vi "PCP Interface Loop.vi"(1 "PCP IO Loop ID":u16, 11 "error in (no error)":errorcluster) -> ()   [LabVIEW 2011]
uses:
  PCP Commands.ctl
  <vilib>/Instr/_visa.llb/VISA Flush IO Buffer Mask.ctl
  emi Lib/System 01/0 - General/App/Loop control 2/Private/_emi_ SMLoop start condition.vi
  emi Lib/System 01/0 - General/App/Loop control 2/Private/_emi_ SMLoop Error Check.vi
  emi Lib/Basic/0 - General/Error/emi_Is Error.vi
  emi Lib/System 01/0 - General/App/Loop control 2/Private/_emi_SMLoop Register new.vi
  emi Lib/System 01/0 - General/S&E reporting/emi_Send S&E Error message.vi
  emi Lib/Basic/0 - General/Error/emi_ Is Error state.vi
  emi Lib/System 01/0 - General/emi_Read System ID.vi
  emi Lib/System 01/0 - General/App/Loop control/Private/_emi_GFV Loop Linking.vi
  emi Lib/System 01/0 - General/App/Loop control/Private/_emi_GFV Loop Enable.vi
  emi Lib/System 01/0 - General/App/Loop control 2/Private/_emi_ SMLoop Restart.vi
  emi Lib/System 01/0 - General/App/Private/_emi_GFV App Close.vi
  emi Lib/System 01/0 - General/App/Loop control 2/Private/_emi_ SMLoop Restart Counter.vi
  emi Lib/System 01/0 - General/App/Loop control/Private/_emi_GFV Loop Running.vi
  emi Lib/System 01/0 - General/Private/_emi_GFV System ID.vi
  emi Lib/System 01/0 - General/S&E reporting/Private/_emi_S&E Q Generator.vi
  emi Lib/System 01/0 - General/App/Loop control/Private/_emi_GFV stop a loop so it can reset.vi
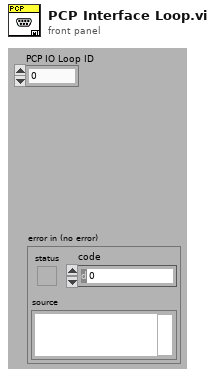
[diagram p1: front panel]
types:
  T1 = typedef "_emi_ SMLoop sates.ctl" = enum16{"Init", "Standby", "Start", "Normal Operation", "Stop", "Error Handling", "End", "Post"}
  T2 = cluster{"Placeholder":bool, "PCP cmd Q":refnum<queue>, "VISA name":refnum<visa-resource-name>}
  T3 = typedef "PCP Command definer.ctl" = cluster{"Action":T4, "n(0)":i32, "d(0.0)":dbl}
  T4 = typedef "PCP Commands.ctl" = enum16{"do not use HE - Help", "RDd - Most used inputs", "RA - All analog inputs", "RE n Reset DO n", "SE n Set DO n", "RP - Get digital inputs", "VA d Set AO A  Motor Volt", "VB d Set AO B  Cable Resistance", "VEr - Get Version", "DYp - Depth counter", "DR - Reset Depth Counter", "DS n Set Depth options(0-3)", "do not use ME - Manual mode enabled", "MD - Manual mode disabled", "ID - Get ID(2001)", "TS - Get Timestamp", "TO d(s)  Set timeout", "do not use LO n Start Loop Mode(1,2)", "AL n RD&LO variation", "ST - Stop Loop Mode"}
  T5 = typedef "VISA Flush IO Buffer Mask.ctl" = u16
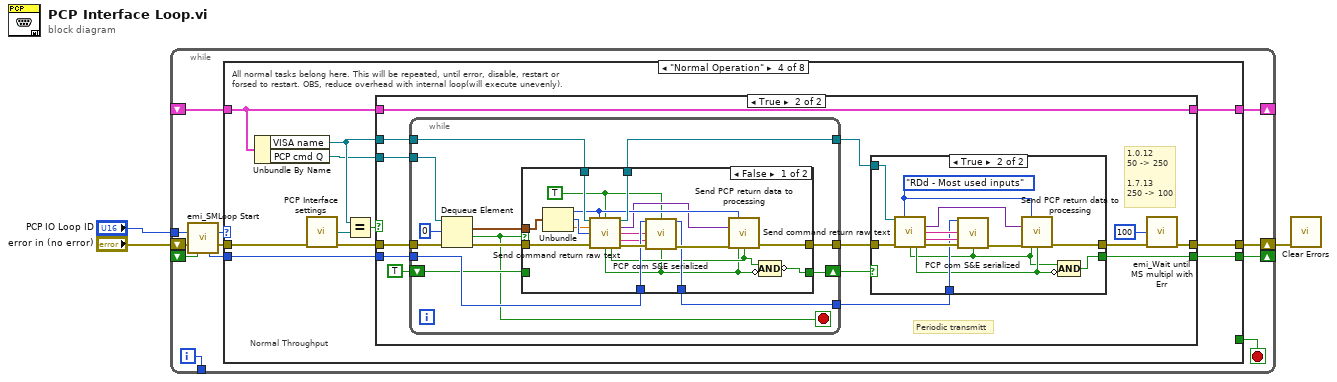
[diagram p0: block diagram]
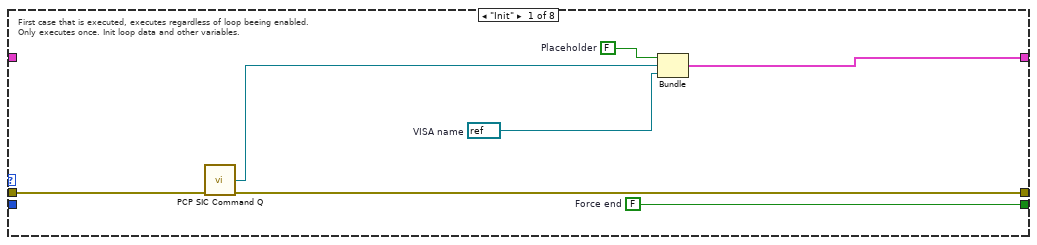
[diagram p2: hidden frame]
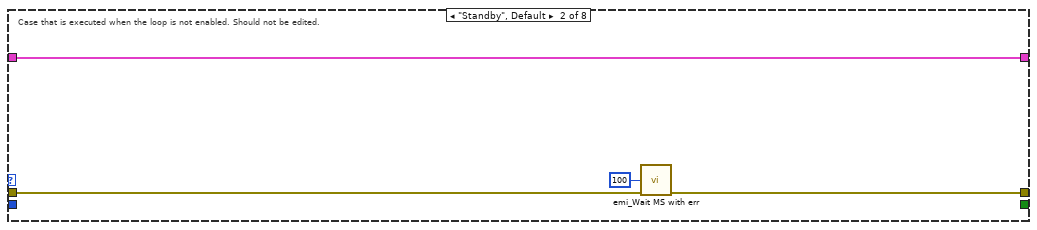
[diagram p3: hidden frame]
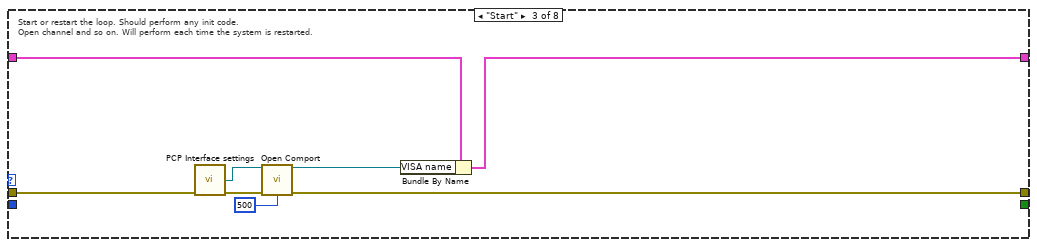
[diagram p4: hidden frame]
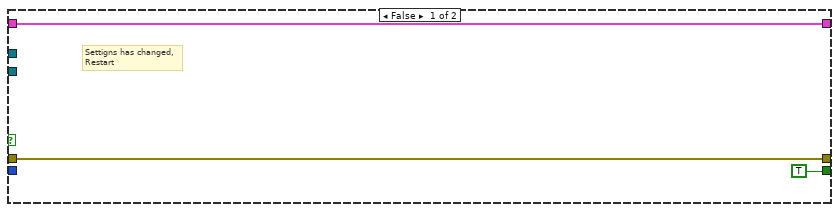
[diagram p5: hidden frame]
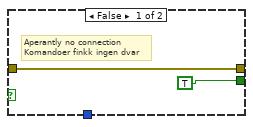
[diagram p6: hidden frame]
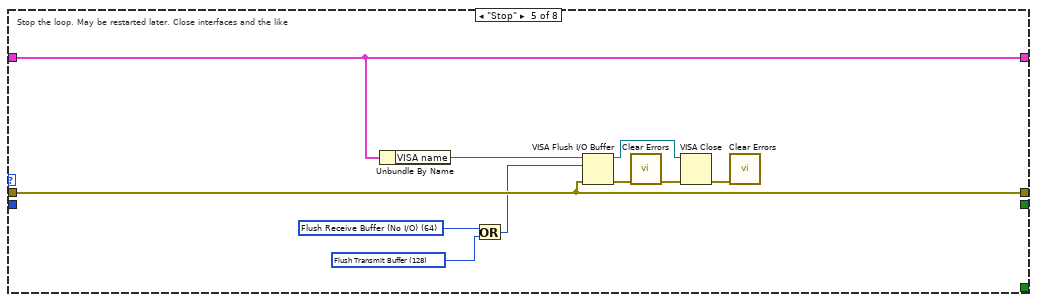
[diagram p8: hidden frame]
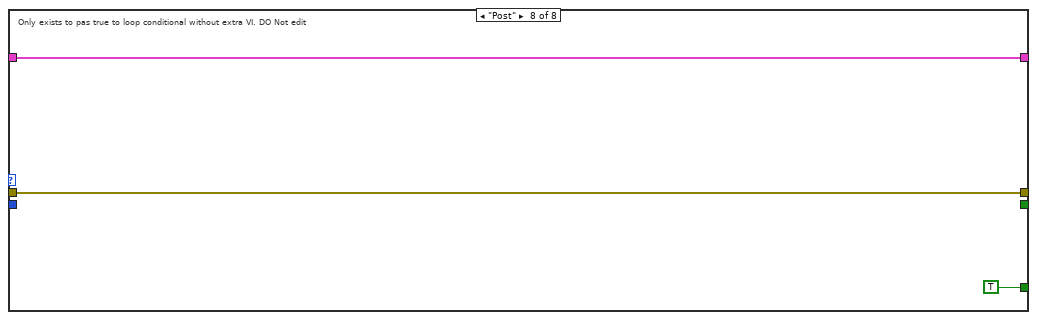
[diagram p11: hidden frame]
diagram:
  n1 = while {
    shift-right: [w15] -> _
    shift-left: _ -> [w11]
    shift-right: [w13] -> w1
    shift-left: "error in (no error)" -> [w9]
    tunnel: [w12] -> _
    shift-right: [w10] -> _
    shift-left: _ -> [w5]
    tunnel: "PCP IO Loop ID" -> [w6]
    i -> [w12]
    stop <- w14 stop-if-true
    n2 = call "emi_SMLoop Start.vi"("Loop ID"=w6, "error in (no error)"=w9, "Force Stop(F)"=w5) -> ("Loop command"=w7:T1, "error out"=w8:errorcluster, "Loop ID out"=w4:i32)  [unwired: 10 in]
    n3 = case shown="\"Normal Operation\"" w7 {
      tunnel: [w18 w23 w30 w43 w122 w125 w126 w129] -> w15
      tunnel: [_ _ _ _ _ _ _ TRUE] -> w14
      tunnel: w8 -> [w16 w25 w33 w45 w119 w124 w127 w130]
      tunnel: [w20 w24 w28 w44 w119 w124 w127 w130] -> w13
      tunnel: w11 -> [_ w23 w34 w42 w122 w125 w126 w129]
      tunnel: [w21 _ _ w41 _ _ _ _] -> w10
      tunnel: w4 -> [_ _ _ w40 _ _ _ _]
      frame "Init" {
        w17 = refnum<visa-resource-name> refnum  # VISA name
        w21 = FALSE  # Force end
        w22 = FALSE  # Placeholder
        # "First case that is executed, executes regardless of loop beeing enabled.\nOnly executes once. Init loop data and other variables."
        n4 = call "PCP SIC Command Q.vi"("error in (no error)"=w16) -> ("PCP cmd Q"=w19:refnum<queue>, "error out"=w20:errorcluster)  [unwired: 13 in]
        n5 = Bundle("Placeholder"=w22, "PCP cmd Q"=w19, "VISA name"=w17) -> (w18:T2)  [unwired: 1 in]
      }
      frame "Standby", Default {
        # "Case that is executed when the loop is not enabled. Should not be edited."
        n6 = call "emi_Wait MS with err.vi"("milliseconds to wait(0)"=u32 100, "error in (no error)"=w25) -> ("error out"=w24:errorcluster)  [unwired: 13 in]
      }
      frame "Start" {
        # "Start or restart the loop. Should perform any init code. \nOpen channel and so on. Will perform each time the system is restarted."
        n7 = call "PCP Interface settings.vi"("error in (no error)"=w33) -> ("PCP VISA  name  out"=w31:refnum<visa-resource-name>, "error out"=w32:errorcluster)  [unwired: 13 in]
        n8 = call "Open Comport.vi"("Comport"=w31, "error in (no error)"=w32, "Reply timeout (300 ms)"=u32 500) -> ("VISA resource name out"=w29:refnum<visa-resource-name>, "error out"=w28:errorcluster)  [unwired: 11 in]
        n9 = Bundle By Name(cluster=w34, "VISA name"=w29) -> (w30:T2)
      }
      frame "Normal Operation" {
        # "Normal Throughput"
        # "All normal tasks belong here. This will be repeated, until error, disable, restart or\nforsed to restart. OBS, reduce overhead with internal loop(will execute unevenly)."
        n10 = Unbundle By Name(w42) -> ("VISA name"=w36:refnum<visa-resource-name>, "PCP cmd Q"=w35:refnum<queue>)
        n11 = call "PCP Interface settings.vi"("error in (no error)"=w45) -> ("PCP VISA  name  out"=w39:refnum<visa-resource-name>, "error out"=w37:errorcluster)  [unwired: 13 in]
        n12 = Equal?(x=w36, y=w39) -> (x = y?=w38:bool)
        n13 = case shown="True" w38 {
          tunnel: w37 -> [w47 w61]
          tunnel: [w46 w62] -> w43
          tunnel: w42 -> [w46 w62]
          tunnel: [TRUE ("Force End") w52] -> w41
          tunnel: [w47 w51] -> w44
          tunnel: w35 -> [_ w60]
          tunnel: w36 -> [_ w59]
          tunnel: w40 -> [_ w58]
          frame False {
            # "Settigns has changed,\nRestart"
          }
          frame True {
            # "1.0.12 \n50 -> 250\n\n1.7.13\n250 -> 100"
            # "Periodic transmitt"
            n14 = while {
              tunnel: w61 -> [w89]
              tunnel: w60 -> [w88]
              tunnel: w59 -> [w85]
              tunnel: w58 -> [w84]
              shift-right: [w82] -> w54
              shift-left: TRUE ("Reply") -> [w83]
              tunnel: [w81] -> w55
              tunnel: [w79] -> w56
              tunnel: [w78] -> w53
              stop <- w80 stop-if-true
              n15 = Dequeue Element(queue=w88, timeout in ms (-1)=0, error in (no error)=w89) -> (element=w86:T3, timed out?=w80:bool, error out=w87:errorcluster)  [unwired: 1 out]
              n16 = case shown="False" w80 {
                tunnel: w87 -> [w105 w110]
                tunnel: [w102 w110] -> w79
                tunnel: w86 -> [w107 _]
                tunnel: w85 -> [w109 w113]
                tunnel: [w108 w113] -> w81
                tunnel: [w91 w112] -> w82
                tunnel: w83 -> [_ w112]
                tunnel: w84 -> [w99 w111]
                tunnel: [w98 w111] -> w78
                frame False {
                  w94 = TRUE ("Periodic")
                  n17 = Unbundle(w107) -> ("Action"=w103:T4, "n(0)"=w106:i32, "d(0.0)"=w104:dbl)
                  n18 = call "Send command return raw text.vi"("VISA resource"=w109, "Action"=w103, "Periodic(F)"=w94, "d(0.0)"=w104, "n(0)"=w106, "error in (no error)"=w105) -> ("VISA resource out"=w108:refnum<visa-resource-name>, "Return Data"=w95:variant, "Return string"=w97:string, "Sendt string"=w96:string, "Reply received"=w92:bool, "Reply Expected"=w93:bool, "error out"=w101:errorcluster)  [unwired: 3 in]
                  n19 = call "PCP com S&E serialized.vi"("Loop ID in"=w99, "Periodic(F)"=w94, "Serialized Receive"=w97, "Serialized send"=w96, "error in (no error)"=w101, "Reply"=w92) -> ("Loop ID out"=w98:u16, "error out"=w100:errorcluster)  [unwired: 8 in]
                  n20 = call "Send PCP return data to processing.vi"("PCP Action"=w103, "Return Data"=w95, "error in"=w100, "Reply Received"=w92, "Reply Expected"=w93) -> ("error out"=w102:errorcluster)  [unwired: 10 in]
                  n21 = Compound Arithmetic op=AND(w93, invert w92) -> (invert w91:bool)
                }
                frame True {
                  # "Timeout"
                }
              }
            }
            n22 = case shown="True" w54 {
              tunnel: w56 -> [w64 w77]
              tunnel: [w64 w76] -> w50
              tunnel: w53 -> [_ w69]
              tunnel: w55 -> [_ w68]
              tunnel: [TRUE w67] -> w52
              frame False {
                # "Aperantly no connection\nKomandoer finkk ingen dvar"
              }
              frame True {
                w75 = PCP_Commands."RDd - Most used inputs" ("Action")
                n23 = call "Send command return raw text.vi"("VISA resource"=w68, "Action"=w75, "error in (no error)"=w77) -> ("Return Data"=w74:variant, "Return string"=w71:string, "Sendt string"=w70:string, "Reply received"=w65:bool, "Reply Expected"=w66:bool, "error out"=w73:errorcluster)  [unwired: 6 in, 1 out]
                n24 = call "PCP com S&E serialized.vi"("Loop ID in"=w69, "Serialized Receive"=w71, "Serialized send"=w70, "error in (no error)"=w73, "Reply"=w65) -> ("error out"=w72:errorcluster)  [unwired: 9 in, 1 out]
                n25 = call "Send PCP return data to processing.vi"("PCP Action"=w75, "Return Data"=w74, "error in"=w72, "Reply Received"=w65, "Reply Expected"=w66) -> ("error out"=w76:errorcluster)  [unwired: 10 in]
                n26 = Compound Arithmetic op=AND(w65, invert w66) -> (w67:bool)
              }
            }
            n27 = call "emi_Wait until MS multipl with Err.vi"("millisecond multiple(0)"=u32 100 ("milliseconds to wait(0)"), "error in (no error)"=w50) -> ("error out"=w51:errorcluster)  [unwired: 13 in]
          }
        }
      }
      frame "Stop" {
        w114 = T5 128 items=["Flush Receive Buffer"=16, "Write Transmit Buffer to Device"=32, "Flush Receive Buffer (No I/O)"=64, "Flush Transmit Buffer"=128] ("Mask")
        w116 = T5 64 items=["Flush Receive Buffer"=16, "Write Transmit Buffer to Device"=32, "Flush Receive Buffer (No I/O)"=64, "Flush Transmit Buffer"=128] ("Mask")
        # "Stop the loop. May be restarted later. Close interfaces and the like"
        n28 = Unbundle By Name(w122) -> ("VISA name"=w118:refnum<visa-resource-name>)
        n29 = Or(x=w116, y=w114) -> (x .or. y?=w115:T5)
        n30 = VISA Flush I/O Buffer(VISA resource name=w118, mask (16)=w115, error in (no error)=w119) -> (VISA resource name out=w117:refnum<visa-resource-name>, error out=w120:errorcluster)
        n31 = call <vilib>:"Clear Errors.vi"("error in (no error)"=w120) -> ("error out"=w121:errorcluster)  [unwired: 6 in]
        n32 = VISA Close(VISA resource name=w117, error in (no error)=w121) -> (error out=w123:errorcluster)
        n33 = call <vilib>:"Clear Errors.vi"("error in (no error)"=w123) -> ()  [unwired: 6 in, 1 out]
      }
      frame "Error Handling" {
        # "Loop automaticaly returns here after error is found. If error is cleared, \nLoop wil continue as normal(if was operative when error."
      }
      frame "End" {
        # "Only executes at application end has. Should performa any action the loop \nneeds to finnish. Executes only once."
      }
      frame "Post" {
        # "Only exists to pas true to loop conditional without extra VI. DO Not edit"
      }
    }
  }
  n34 = call <vilib>:"Clear Errors.vi"("error in (no error)"=w1) -> ()  [unwired: 6 in, 1 out]
